vi "Build.vi"   [LabVIEW 2018, in "Scripts.lvlib"]
uses:
  Scripts.lvlib
  <vilib>/Field R&D Services/Labricator/Toolkit/Labricator.lvlib
panel:
  # "Overview: Builds all Source Distribution specifications for this project\nRequirements: LabVIEW, Application Builder\nInstructions: Run this VI.\n\nThis VI builds all of the build specifications for this project. Any version of LabVIEW that supports projects and the Application Builder API can be used."
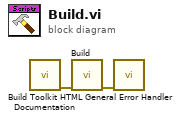
[diagram p0: block diagram]
diagram:
  n1 = call "Build Toolkit HTML Documentation.vi"() -> ("Error Out"=w1:errorcluster)  [unwired: 11 in]
  n2 = call <vilib>:"Build.vi"("Error In"=w1) -> ("Error Out"=w2:errorcluster)  [unwired: 10 in]
  n3 = call <vilib>:"General Error Handler.vi"("error in (no error)"=w2) -> ()  [unwired: 10 in, 5 out]
